vi "SysParamRef.vi"(7 "Init":bool, 9 "System Up time":refnum<vi>, 11 "Unit Add":refnum<vi>) -> (1 "System Up time out":refnum<vi>, 3 "Unit Add out":refnum<vi>)   [LabVIEW 2010]
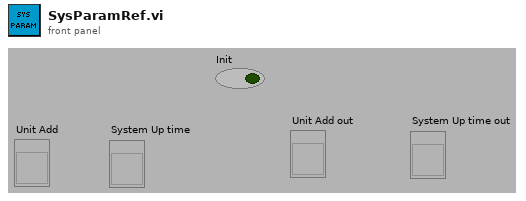
[diagram p1: front panel]
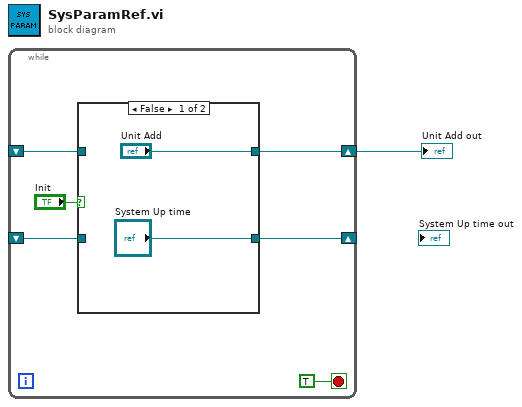
[diagram p0: block diagram]
diagram:
  n1 = while {
    shift-right: [w6] -> w1
    shift-left: _ -> [w5]
    shift-right: [w3] -> _
    shift-left: _ -> [w2]
    stop <- TRUE stop-if-true
    n2 = case shown="False" "Init" {
      tunnel: ["Unit Add" w11] -> w6
      tunnel: w5 -> [_ w11]
      tunnel: ["System Up time" w10] -> w3
      tunnel: w2 -> [_ w10]
      frame False {
      }
      frame True {
      }
    }
  }
  "Unit Add out" <- w1
